vi "Discover Gantry.vi"(0 "Session In":refnum<visa-resource-name>="COM5", 5 "error in":errorcluster {"code" format="%.0x"}, 9 "Close Session(t)":bool=TRUE) -> (10 "Gantry Present(t)":bool=TRUE, 12 "TestBench_ID":string="WAM_PROD_TEST-1", 13 "concatenated string":string="#INST: Gantry#Address COM5#Manufacturer Zaber#Model X-MCC4 (rev 1)#SN 81246#Ver (FW) 7.21 (DR) 1.5", 14 "Session Out":refnum<visa-resource-name>="COM5", 15 "Mfr":string="Zaber", 16 "Model":string="X-MCC4 (rev 1)", 17 "Ver":string="(FW) 7.21 (DR) 1.5", 18 "SN":string="81246", 19 "error out":errorcluster)   [LabVIEW 2018]
uses:
  Sequence Globals.vi
  Instruments/Zaber Gantry/Zaber Labview Driver/Zaber A Series.lvlib
  <vilib>/Utility/file.llb/Read Delimited Spreadsheet (string).vi
panel:
  out "ok?(t)":bool
  out "FH_NOT(T)":bool=TRUE
  out "S/N":string="81246"
  out "Instrument Driver Revision":string="1.5"
  out "Instrument Firmware Revision":string="7.21"
  out "Pass Self-Test(t)":bool=TRUE
  out "Peripheral ID":i32=70140
  out "Device ID":i32=30342
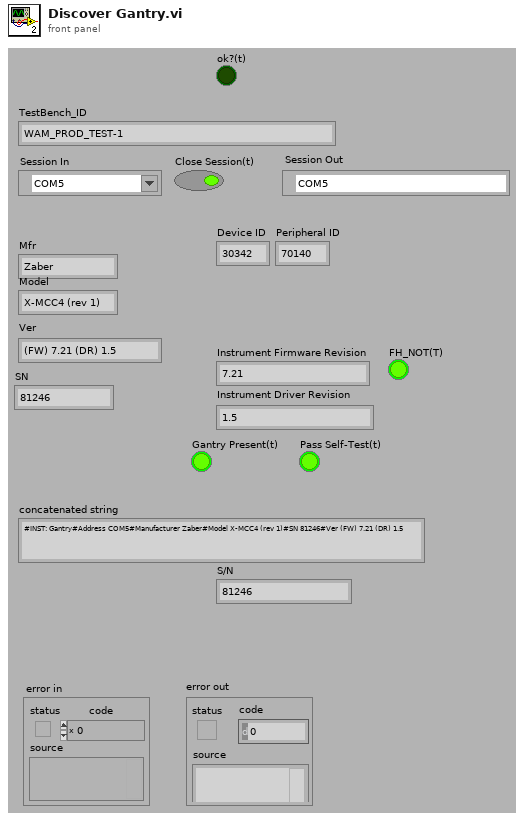
[diagram p1: front panel]
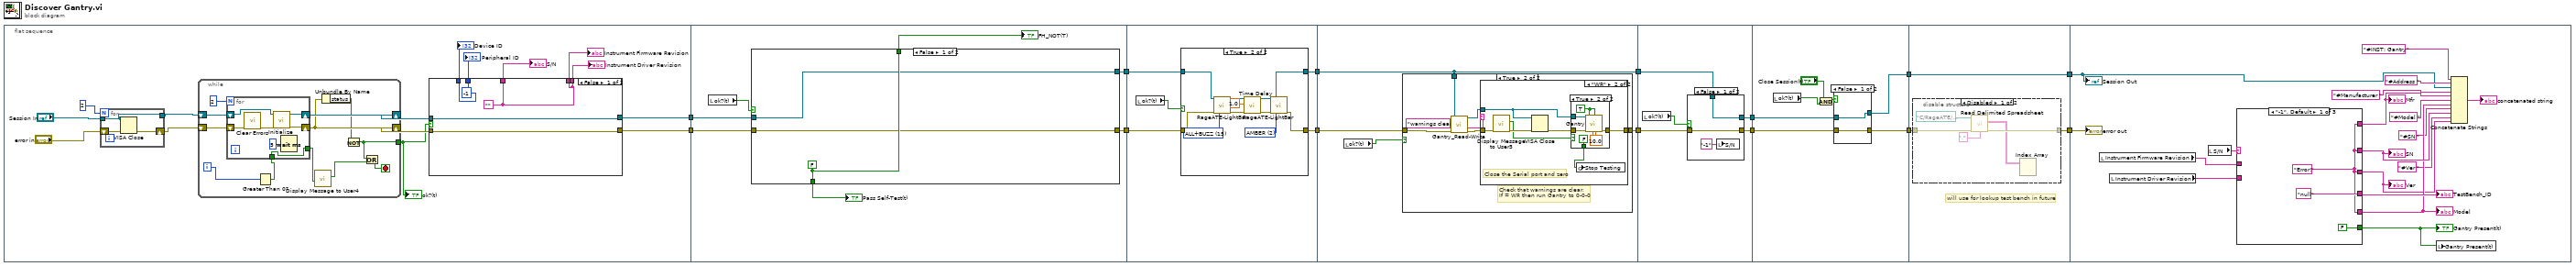
[diagram p0: block diagram]
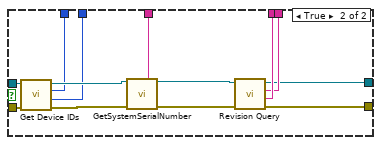
[diagram p2: hidden frame]
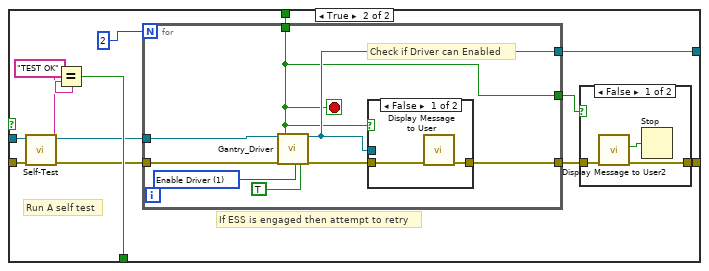
[diagram p3: hidden frame]
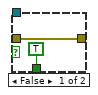
[diagram p9: hidden frame]
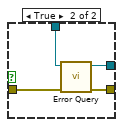
[diagram p10: hidden frame]
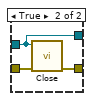
[diagram p11: hidden frame]
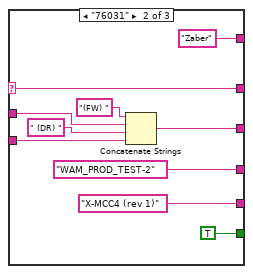
[diagram p13: hidden frame]
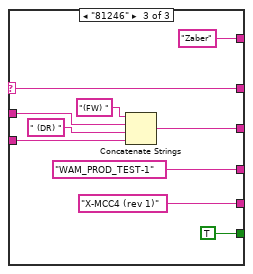
[diagram p14: hidden frame]
diagram:
  n1 = flat-sequence {
    tunnel: [w24] -> w14
    tunnel: [w21] -> w13
    tunnel: w14 -> [w71]
    tunnel: w13 -> [w72]
    tunnel: [w74] -> w8
    tunnel: [w73] -> w6
    tunnel: w8 -> [w109]
    tunnel: [w108] -> w7
    tunnel: w6 -> [w110]
    tunnel: [w111] -> w5
    tunnel: w7 -> [w125]
    tunnel: w5 -> [w127]
    tunnel: [w126] -> w12
    tunnel: [w125] -> w11
    tunnel: [w155] -> w10
    tunnel: [w154] -> w9
    tunnel: w12 -> [w156]
    tunnel: w11 -> [w153]
    tunnel: [w170] -> w4
    tunnel: [w169] -> w2
    tunnel: w9 -> [w167]
    tunnel: w10 -> [w168]
    tunnel: w4 -> [w176]
    tunnel: [w177] -> w3
    tunnel: w2 -> [w178]
    tunnel: [w178] -> w1
    tunnel: w3 -> [w187]
    tunnel: w1 -> [w186]
    frame #0 {
      n2 = for {
        N: 2 -> [_]
        tunnel: "Session In" -> [w66]
        shift-right: [w67] -> w15
        shift-left: "error in" -> [w68]
        tunnel: [w66] -> w17
        n3 = VISA Close(VISA resource name=w66, error in (no error)=w68) -> (error out=w67:errorcluster)
      }
      n4 = while {
        shift-right: [w58] -> w28
        shift-left: w17 -> [w56]
        shift-right: [w54] -> w29
        shift-left: w15 -> [w55]
        tunnel: [w51] -> w16
        i -> [w50]
        stop <- w52 stop-if-true
        n5 = Greater Than 0?(x=w50) -> (x > 0?=w48:bool)
        n6 = for {
          N: 2 -> [_]
          shift-right: [w64] -> w58
          shift-left: w56 -> [w60]
          shift-right: [w65] -> w54
          shift-left: w55 -> [w62]
          tunnel: w48 -> [w59]
          tunnel: [w59] -> w47
          n7 = call <vilib>:"Clear Errors.vi"("error in (no error)"=w62) -> ("error out"=w61:errorcluster)  [unwired: 5 in, 1 out]
          n8 = call "Initialize.vi"("error in (no error)"=w61, "VISA resource name"=w60) -> ("error out"=w65:errorcluster, "VISA resource name out"=w64:refnum<visa-resource-name>)  [unwired: 8 in]
          n9 = Wait (ms)(milliseconds to wait=u32 5) -> ()  [unwired: 1 out]
        }
        n10 = call "Display Message to User4"("Enable"=w47) -> ("QUIT"=w49:bool)  [unwired: 9 in, 1 out]
        n11 = Unbundle By Name(w54) -> ("status"=w53:bool)
        n12 = Not(x=w53) -> (.not. x?=w51:bool)
        n13 = Or(x=w51, y=w49) -> (x .or. y?=w52:bool)
      }
      "ok?(t)" <- w16
      n14 = case shown="False" w16 {
        tunnel: w29 -> [w33 w44]
        tunnel: w28 -> [w32 w43]
        tunnel: [w31 w42] -> w27
        tunnel: [w30 w41] -> w26
        tunnel: [w30 w40] -> w25
        tunnel: [w33 w37] -> w24
        tunnel: [w31 w36] -> w23
        tunnel: [w31 w35] -> w22
        tunnel: [w32 w34] -> w21
        frame False {
          w30 = -1 ("Peripheral ID")
          w31 = ""
        }
        frame True {
          n15 = call "Get Device IDs.vi"("error in (no error)"=w44, "VISA resource name"=w43) -> ("error out"=w46:errorcluster, "Peripheral ID"=w40:i32, "Device ID"=w41:i32, "VISA resource name out"=w45:refnum<visa-resource-name>)  [unwired: 6 in]
          n16 = call "GetSystemSerialNumber.vi"("VISA resource name"=w45, "error in (no error)"=w46) -> ("S/N"=w42:string, "VISA resource name out"=w38:refnum<visa-resource-name>, "error out"=w39:errorcluster)  [unwired: 11 in]
          n17 = call "Revision Query.vi"("error in (no error)"=w39, "VISA resource name"=w38) -> ("error out"=w37:errorcluster, "Instrument Firmware Revision"=w36:string, "Instrument Driver Revision"=w35:string, "VISA resource name out"=w34:refnum<visa-resource-name>)  [unwired: 6 in]
        }
      }
      "Device ID" <- w26
      "Peripheral ID" <- w25
      "Instrument Firmware Revision" <- w23
      "Instrument Driver Revision" <- w22
      "S/N" <- w27
    }
    frame #1 {
      n18 = local read "ok?(t)"() -> (w69:bool)
      n19 = case shown="False" w69 {
        tunnel: [w78 w91] -> w75
        tunnel: [w76 w85] -> w74
        tunnel: [w77 w83] -> w73
        tunnel: w72 -> [w76 w81]
        tunnel: w71 -> [w77 w80]
        tunnel: [w78 w79] -> w70
        frame False {
          w78 = FALSE
        }
        frame True {
          # "If ESS is engaged then attempt to retry"
          # "Run A self test"
          n20 = call "Self-Test.vi"("error in (no error)"=w80, "VISA resource name"=w81) -> ("error out"=w88:errorcluster, "Self-Test Result Message"=w89:string, "VISA resource name out"=w87:refnum<visa-resource-name>)  [unwired: 7 in]
          n21 = Equal?(x=w89, y="TEST OK") -> (x = y?=w91:bool)
          n22 = for {
            N: 2 -> [_]
            tunnel: w88 -> [w103]
            tunnel: w87 -> [w102]
            tunnel: [w99] -> w84
            tunnel: [w98] -> w85
            tunnel: [w96] -> w82
            tunnel: [w96] -> w79
            stop <- w96 stop-if-true
            w101 = u16 1 items=["Disable Driver", "Enable Driver", "Read Driver Status"] ("Driver-Func")
            # "Check if Driver can Enabled"
            n23 = call "Gantry_Driver.vi"("VISA resource name"=w102, "error in (no error)"=w103, "Driver-Func"=w101, "Close Serial"=TRUE) -> ("FH_NOT(T)"=w96:bool, "VISA resource name out"=w98:refnum<visa-resource-name>, "error out"=w100:errorcluster)  [unwired: 12 in, 1 out]
            n24 = case shown="False" w96 {
              tunnel: w98 -> [_ _]
              tunnel: w100 -> [w104 w106]
              tunnel: [w105 w106] -> w99
              frame False {
                n25 = call "Display Message to User"("error in (no error)"=w104) -> ("error out"=w105:errorcluster)  [unwired: 9 in, 1 out]
              }
              frame True {
              }
            }
          }
          n26 = case shown="False" w82 {
            tunnel: w84 -> [w94 w95]
            tunnel: [w93 w95] -> w83
            frame False {
              n27 = call "Display Message to User2"("error in (no error)"=w94) -> ("error out"=w93:errorcluster, "OK"=w92:bool)  [unwired: 9 in]
              n28 = Stop(stop? (T)=w92) -> ()
            }
            frame True {
            }
          }
        }
      }
      "Pass Self-Test(t)" <- w75
      "FH_NOT(T)" <- w70
    }
    frame #2 {
      n29 = local read "ok?(t)"() -> (w107:bool)
      n30 = case shown="True" w107 {
        tunnel: [w112 w123] -> w111
        tunnel: w110 -> [w112 w122]
        tunnel: w109 -> [w113 w121]
        tunnel: [w113 w120] -> w108
        frame False {
        }
        frame True {
          w118 = u32 2 items=["RED"=1, "AMBER"=2, "GREEN"=4, "ALL"=7, "BUZZ"=8, "RED+BUZZ"=9, "ALL+BUZZ"=15] ("Select")
          w119 = u32 15 items=["RED"=1, "AMBER"=2, "GREEN"=4, "ALL"=7, "BUZZ"=8, "RED+BUZZ"=9, "ALL+BUZZ"=15] ("Select")
          n31 = call "RageATE-LightBar.vi"("VISA resource name"=w121, "error in"=w122, "Select"=w119) -> ("VISA resource name out"=w117:refnum<visa-resource-name>, "error out"=w115:errorcluster)  [unwired: 10 in, 1 out]
          n32 = call "Time Delay"("error in (no error)"=w115, "Delay Time (s)"=1.0) -> ("error out"=w116:errorcluster)  [unwired: 9 in]
          n33 = call "RageATE-LightBar.vi"("VISA resource name"=w117, "error in"=w116, "Select"=w118) -> ("VISA resource name out"=w120:refnum<visa-resource-name>, "error out"=w123:errorcluster)  [unwired: 10 in, 1 out]
        }
      }
    }
    frame #3 {
      n34 = local read "ok?(t)"() -> (w124:bool)
      n35 = case shown="True" w124 {
        tunnel: w127 -> [w128 w134]
        tunnel: [w128 w130] -> w126
        tunnel: w125 -> [_ w129]
        frame False {
        }
        frame True {
          # "Check that warnings are clear,\nIf = WR then run Gantry to 0-0-0"
          n36 = call "Gantry_Read-Write.vi"("VISA resource name"=w129, "Command"="warnings clear", "error in (no error)"=w134) -> ("VISA resource name out"=w131:refnum<visa-resource-name>, "Warning Flags"=w133:string, "error out"=w132:errorcluster)  [unwired: 6 in, 4 out]
          n37 = case shown="\"WR\"" w133 {
            tunnel: w132 -> [w136 w139]
            tunnel: w131 -> [_ w142]
            tunnel: [w136 w143] -> w130
            frame "False", Default {
            }
            frame "WR" {
              # "Close the Serial port and zero"
              n38 = call "Display Message to User3"("error in (no error)"=w139) -> ("error out"=w140:errorcluster, "OK"=w138:bool)  [unwired: 9 in]
              n39 = VISA Close(VISA resource name=w142, error in (no error)=w140) -> (error out=w141:errorcluster)
              n40 = case shown="True" w138 {
                tunnel: [w145 w151] -> w143
                tunnel: w142 -> [_ w148]
                tunnel: w141 -> [w145 w147]
                tunnel: [TRUE ("Stop Testing") FALSE ("Stop Testing")] -> w137
                frame False {
                }
                frame True {
                  w150 = 10.0 ("z ref")
                  w149 = TRUE ("Use manual(t)")
                  n41 = call "Gantry.vi"("COMPORT"=w148, "error in (no error)"=w147, "Use manual(t)"=w149, "z ref"=w150, "Write(reads antenna co-ords when off)"=w149, "z"=w150) -> ("error out"=w151:errorcluster)  [unwired: 13 in]
                }
              }
              n42 = global write "Sequence Globals.vi" "Stop Testing"(w137) -> ()
            }
          }
        }
      }
    }
    frame #4 {
      n43 = local read "ok?(t)"() -> (w152:bool)
      n44 = case shown="False" w152 {
        tunnel: w156 -> [w158 w163]
        tunnel: [w158 w162] -> w155
        tunnel: [w159 w161] -> w154
        tunnel: w153 -> [w159 w160]
        frame False {
          n45 = local write "S/N"("-1" ("S/N")) -> ()
        }
        frame True {
          n46 = call "Error Query.vi"("error in (no error)"=w163, "VISA resource name"=w160) -> ("error out"=w162:errorcluster, "VISA resource name out"=w161:refnum<visa-resource-name>)  [unwired: 6 in, 2 out]
        }
      }
    }
    frame #5 {
      n47 = local read "ok?(t)"() -> (w164:bool)
      n48 = And(x="Close Session(t)", y=w164) -> (x .and. y?=w166:bool)
      n49 = case shown="False" w166 {
        tunnel: w168 -> [w172 w175]
        tunnel: [w172 w174] -> w170
        tunnel: w167 -> [w171 w173]
        tunnel: [w171 w173] -> w169
        frame False {
        }
        frame True {
          n50 = call "Close.vi"("error in (no error)"=w175, "VISA resource name"=w173) -> ("error out"=w174:errorcluster)  [unwired: 9 in]
        }
      }
    }
    frame #6 {
      # "will use for lookup test bench in future"
      n51 = disable-structure shown="Disabled" {
        disable-tunnel: [w183 w184] -> w177
        disable-tunnel: w176 -> [w182 w184]
        frame Disabled {
          n52 = call-poly <vilib>:"Read Delimited Spreadsheet.vi"("file path (dialog if empty)"=path "C:/RageATE/Automated Tests/Tetra WAM/PRODUCTION/setup files/TestBenches.txt", "error in (no error)"=w182, "delimiter (\\t)"="," ("delimiter (\\t)")) -> ("all rows"=w180:string[][], "error out"=w183:errorcluster)  [unwired: 7 in, 4 out]
          n53 = Index Array(array=w180) -> ()  [unwired: 2 in, 1 out]
        }
        frame Enabled {
        }
      }
    }
    frame #7 {
      n54 = local read "Instrument Firmware Revision"() -> (w201:string)
      n55 = local read "Instrument Driver Revision"() -> (w202:string)
      n56 = local read "S/N"() -> (w200:string)
      n57 = case shown="\"-1\", Default" w200 {
        selector: w200 -> [_ w206 w216]
        tunnel: [w203 "Zaber" ("string") "Zaber" ("string")] -> w195
        tunnel: [w203 "X-MCC4 (rev 1)" ("string") "X-MCC4 (rev 1)" ("string")] -> w196
        tunnel: [w203 w206 w216] -> w197
        tunnel: [w203 w213 w223] -> w194
        tunnel: w201 -> [_ w212 w222]
        tunnel: w202 -> [_ w209 w219]
        tunnel: [FALSE ("Gantry Present(t)") TRUE TRUE] -> w198
        tunnel: ["null" ("string") "WAM_PROD_TEST-2" ("string") "WAM_PROD_TEST-1" ("string")] -> w199
        frame "-1", Default {
          w203 = "Error!" ("string")
        }
        frame "76031" {
          n58 = Concatenate Strings("(FW) " ("string"), w212, " (DR) " ("string"), w209) -> (w213:string)
        }
        frame "81246" {
          n59 = Concatenate Strings("(FW) " ("string"), w222, " (DR) " ("string"), w219) -> (w223:string)
        }
      }
      "Ver" <- w194
      "Mfr" <- w195
      "Model" <- w196
      "SN" <- w197
      "Gantry Present(t)" <- w198
      "TestBench_ID" <- w199
      n60 = local write "Gantry Present(t)"(w198) -> ()
      n61 = Concatenate Strings("#INST: Gantry" ("string"), "#Address " ("string"), w186, "#Manufacturer ", w195, "#Model ", w196, "#SN " ("string"), w197, "#Ver " ("string"), w194) -> (→"concatenated string":string)
      "Session Out" <- w186
      "error out" <- w187
    }
  }
